vi "Load config.vi"(7 "Main VI":refnum<vi>, 8 "error in (no error)":errorcluster, 10 "Graph_refs":T1, 11 "configuration file path":path) -> (0 "error out":errorcluster)   [LabVIEW 2025]
uses:
  Scope/controls/Graph_references.ctl
  Scope/controls/graph_controls.ctl
  <vilib>/Utility/config.llb/NI_LVConfig.lvlib
  <userlib>/_OpenG.lib/variantconfig/variantconfig.llb/openg_variant_configuration_file.lvlib
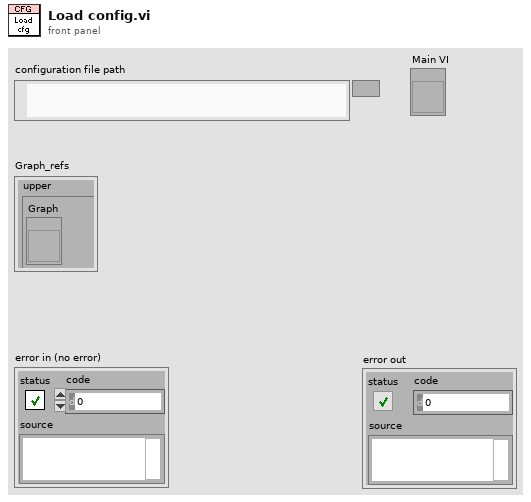
[diagram p1: front panel]
types:
  T1 = typedef "Graph_references.ctl" = cluster{"upper":T2, "lower":T2, "Freq graph":refnum<vi>, "Adaptive FF graph":refnum<vi>}
  T2 = typedef "graph_controls.ctl" = cluster{"Graph":refnum<vi>, "Time btn":refnum<vi>, "Amplitude btn":refnum<vi>, "Chart":refnum<vi>}
  T3 = typedef "NI_LVConfig.lvlib/Config Data RefNum.ctl" = refnum<k1>
  T4 = typedef "Plot visibility.ctl" = cluster{"Visible":bool[], "Name":string}
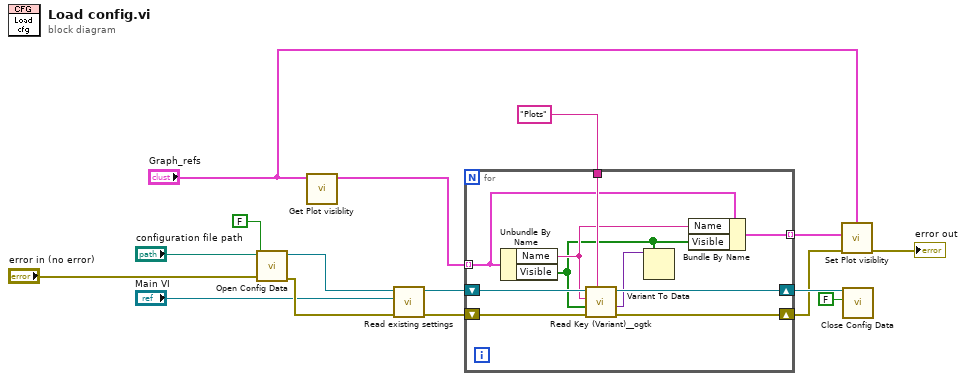
[diagram p0: block diagram]
diagram:
  n1 = call <vilib>:"Open Config Data.vi"("error in (no error)"="error in (no error)", "create file if necessary (T)"=FALSE, "configuration file path"="configuration file path") -> ("error out"=w14:errorcluster, "refnum"=w16:T3)  [unwired: 6 in, 1 out]
  n2 = call "Get Plot visiblity.vi"("Graph_refs"="Graph_refs") -> ("Plot visibility"=w13:T4[])  [unwired: 10 in]
  n3 = call "Read existing settings.vi"("error in (no error)"=w14, "VI ref"="Main VI", "refnum"=w16) -> ("error out"=w11:errorcluster, "refnum out"=w12:T3)  [unwired: 7 in]
  n4 = for {
    tunnel: w13 -> [w19] mode=indexing
    shift-right: [w24] -> w10
    shift-left: w12 -> [w26]
    tunnel: "Plots" -> [w23]
    shift-right: [w22] -> w4
    shift-left: w11 -> [w25]
    tunnel: [w17] -> w6 mode=indexing
    n5 = Unbundle By Name(w19) -> ("Name"=w20:string, "Visible"=w18:bool[])
    n6 = call <userlib>:"Read Key (Variant)__ogtk.vi"("section"=w23, "error in (no error)"=w25, "type"=w18, "key (optional)"=w20, "refnum"=w26) -> ("error out"=w22:errorcluster, "key-value"=w21:variant, "refnum out"=w24:T3)  [unwired: 3 in, 1 out]
    n7 = Variant To Data(type=w18, Variant=w21) -> ()  [unwired: 1 in, 2 out]
    n8 = Bundle By Name(cluster=w19, "Name"=w20, "Visible"=w18) -> (w17:T4)
  }
  n9 = call "Set Plot visiblity.vi"("error in (no error)"=w4, "Plot visibility"=w6, "Graph_refs"="Graph_refs") -> ("error out"=→"error out":errorcluster)  [unwired: 8 in]
  n10 = call <vilib>:"Close Config Data.vi"("write file if changed (T)"=FALSE, "refnum"=w10) -> ()  [unwired: 8 in, 2 out]
